vi "MXG_Set_ARB_State.vi"(8 "error in":errorcluster, 10 "ARB State":string(combo)="ON", 11 "VISA resource name":refnum<visa-resource-name>) -> (0 "error out":errorcluster, 3 "VISA resource name":refnum<visa-resource-name>)   [LabVIEW 2016]
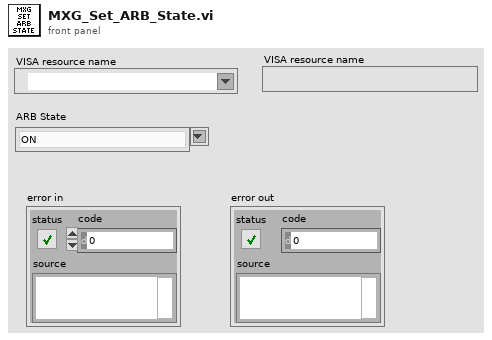
[diagram p1: front panel]
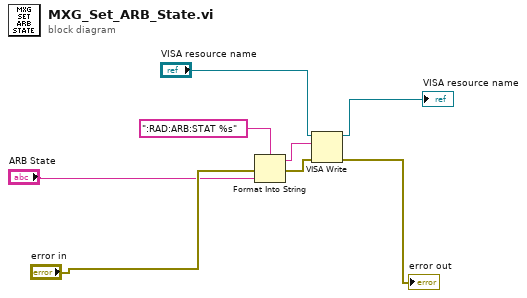
[diagram p0: block diagram]
diagram:
  n1 = Format Into String(format string=":RAD:ARB:STAT %s", error in="error in", "ARB State") -> (resulting string=w3:string, error out=w6:errorcluster)  [unwired: 1 in]
  n2 = VISA Write(VISA resource name="VISA resource name", write buffer=w3, error in (no error)=w6) -> (VISA resource name out=→"VISA resource name":refnum<visa-resource-name>, error out=→"error out":errorcluster)  [unwired: 1 out]
